vi "(Loop) Chamber.vi"   [LabVIEW 2017]
uses:
  Controls/(Ctrl) State_Chamber Loop.ctl
  Controls/(Ctrl) State_Chamber.ctl
  Variables/(Var) System.vi
  Variables/(Var) Chamber.vi
types:
  T1 = typedef "(Ctrl) State_Chamber Loop.ctl" = enum16{"Open", "Rx", "Tx", "Close"}
  T2 = typedef "(Ctrl) State_Chamber.ctl" = enum16{"Open", "Rx : Temp", "Rx : Target Temp", "Rx : State", "Tx : ON-OFF", "Tx : Target Temp", "Tx : Time Set", "Close"}
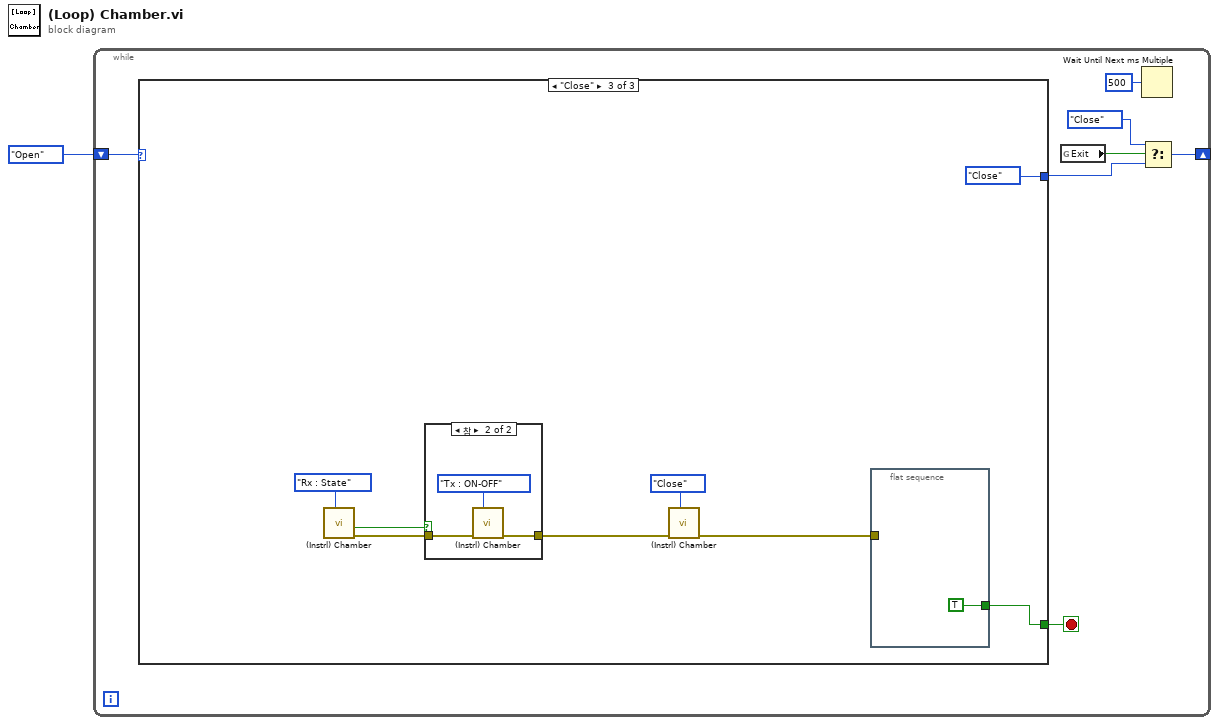
[diagram p0: block diagram]
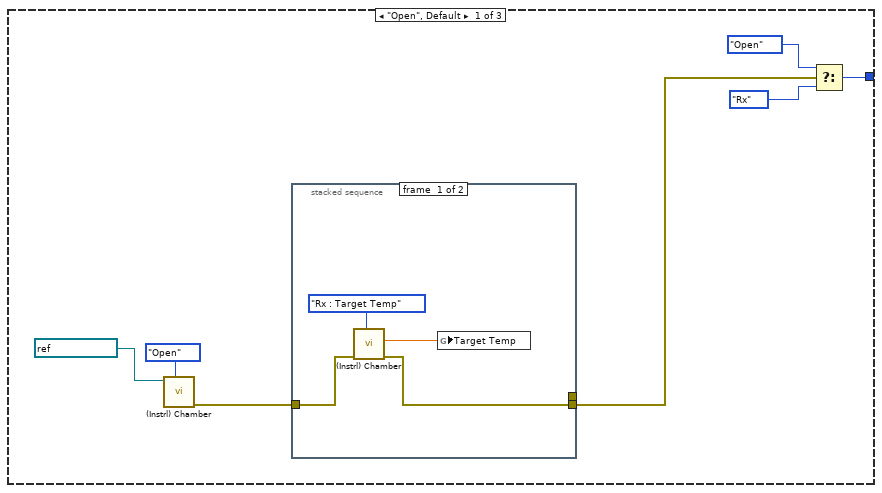
[diagram p2: hidden frame]
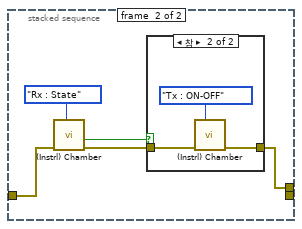
[diagram p3: hidden frame]
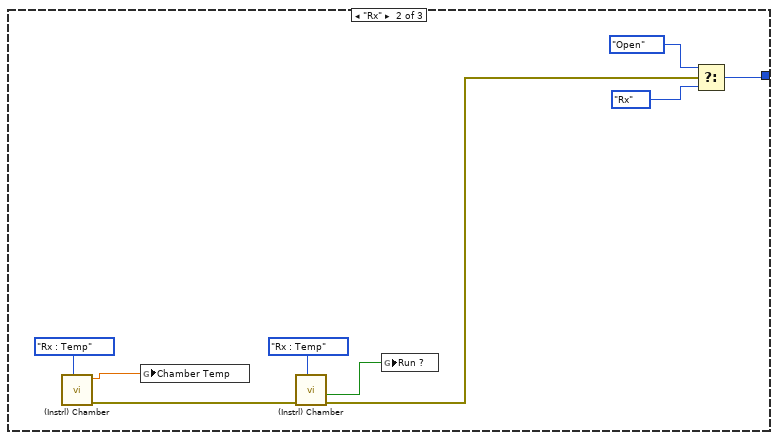
[diagram p5: hidden frame]
diagram:
  n1 = while {
    shift-right: [w3] -> _
    shift-left: (Ctrl)_State_Chamber_Loop."Open" ("State") -> [w8]
    stop <- w2 stop-if-true
    n2 = case shown="\"Close\"" w8 {
      tunnel: [w12 w34 (Ctrl)_State_Chamber_Loop."Close" ("State")] -> w5
      tunnel: [_ _ w39] -> w2
      frame "Open", Default {
        n3 = call "(Instrl) Chamber.vi"("State"=(Ctrl)_State_Chamber."Open", "Com"=refnum<visa-resource-name> "COM7") -> ("error out"=w13:errorcluster)  [unwired: 6 in, 3 out]
        n4 = stacked-sequence {
          tunnel: w13 -> [w19 w24]
          tunnel: [w17 _] -> w11
          tunnel: [_ w21] -> _
          frame #0 {
            n5 = call "(Instrl) Chamber.vi"("State"=(Ctrl)_State_Chamber."Rx : Target Temp", "error in (no error)"=w19) -> ("error out"=w17:errorcluster, "Target Temp"=w16:dbl)  [unwired: 6 in, 2 out]
            n6 = global write "(Var) Chamber.vi" "Target Temp"(w16) -> ()
          }
          frame #1 {
            n7 = call "(Instrl) Chamber.vi"("State"=(Ctrl)_State_Chamber."Rx : State", "error in (no error)"=w24) -> ("error out"=w22:errorcluster, "Run ?"=w20:bool)  [unwired: 6 in, 2 out]
            n8 = case shown="참" w20 {
              tunnel: w22 -> [w25 w28]
              tunnel: [w25 w26] -> w21
              frame False {
              }
              frame True {
                n9 = call "(Instrl) Chamber.vi"("State"=(Ctrl)_State_Chamber."Tx : ON-OFF", "error in (no error)"=w28) -> ("error out"=w26:errorcluster)  [unwired: 6 in, 3 out]
              }
            }
          }
        }
        n10 = Select(t=(Ctrl)_State_Chamber_Loop."Open" ("State"), s=w11, f=(Ctrl)_State_Chamber_Loop."Rx" ("State")) -> (s? t:f=w12:T1)
      }
      frame "Rx" {
        n11 = call "(Instrl) Chamber.vi"("State"=(Ctrl)_State_Chamber."Rx : Temp") -> ("error out"=w31:errorcluster, "Chamber Temp"=w33:dbl)  [unwired: 7 in, 2 out]
        n12 = global write "(Var) Chamber.vi" "Chamber Temp"(w33) -> ()
        n13 = call "(Instrl) Chamber.vi"("State"=(Ctrl)_State_Chamber."Rx : Temp", "error in (no error)"=w31) -> ("error out"=w30:errorcluster, "Run ?"=w29:bool)  [unwired: 6 in, 2 out]
        n14 = global write "(Var) Chamber.vi" "Run ?"(w29) -> ()
        n15 = Select(t=(Ctrl)_State_Chamber_Loop."Open" ("State"), s=w30, f=(Ctrl)_State_Chamber_Loop."Rx" ("State")) -> (s? t:f=w34:T1)
      }
      frame "Close" {
        n16 = call "(Instrl) Chamber.vi"("State"=(Ctrl)_State_Chamber."Rx : State") -> ("error out"=w44:errorcluster, "Run ?"=w45:bool)  [unwired: 7 in, 2 out]
        n17 = case shown="참" w45 {
          tunnel: w44 -> [w47 w50]
          tunnel: [w47 w48] -> w42
          frame False {
          }
          frame True {
            n18 = call "(Instrl) Chamber.vi"("State"=(Ctrl)_State_Chamber."Tx : ON-OFF", "error in (no error)"=w50) -> ("error out"=w48:errorcluster)  [unwired: 6 in, 3 out]
          }
        }
        n19 = call "(Instrl) Chamber.vi"("State"=(Ctrl)_State_Chamber."Close", "error in (no error)"=w42) -> ("error out"=w40:errorcluster)  [unwired: 6 in, 3 out]
        n20 = flat-sequence {
          tunnel: w40 -> [_]
          tunnel: [TRUE] -> w39
          frame #0 {
          }
        }
      }
    }
    n21 = global read "(Var) System.vi" "Exit"() -> (w7:bool)
    n22 = Wait Until Next ms Multiple(millisecond multiple=u32 500 ("대기 시간 (ms)")) -> ()  [unwired: 1 out]
    n23 = Select(t=(Ctrl)_State_Chamber_Loop."Close" ("State"), s=w7, f=w5) -> (s? t:f=w3:T1)
  }
